vi "Update CW Indicators.vi"(8 "error  in":errorcluster, 10 "Car Wash Steps":string[][](array[string]), 11 "Position Correct?":bool) -> (0 "error out":errorcluster, 3 "Car Wash Indicators":T1)   [LabVIEW 2020]
uses:
  Controls/Car Wash Indicators.ctl
  7d301b4d-829d-4e45-9de8-334e8fe51d28.vi
  <vilib>/Comparison/Equal/Equal Functor/Equal Functor.lvclass
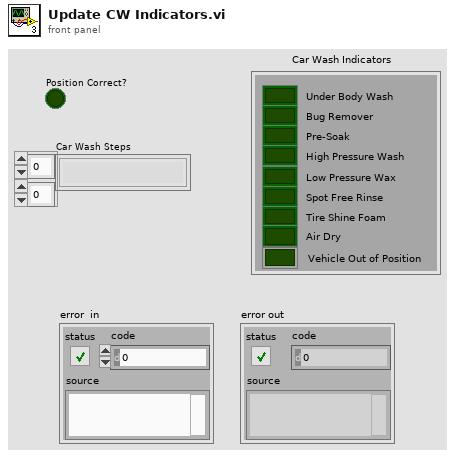
[diagram p1: front panel]
types:
  T1 = typedef "Car Wash Indicators.ctl" = cluster{"Under Body Wash":bool, "Bug Remover":bool, "Pre-Soak":bool, "High Pressure Wash":bool, "Low Pressure Wax":bool, "Spot Free Rinse":bool, "Tire Shine Foam":bool, "Air Dry":bool, "Vehicle Out of Position":bool}
  T2 = cluster{"Car Wash Indicators[0]":bool, "Car Wash Indicators[1]":bool, "Car Wash Indicators[2]":bool, "Car Wash Indicators[3]":bool, "Car Wash Indicators[4]":bool, "Car Wash Indicators[5]":bool, "Car Wash Indicators[6]":bool, "Car Wash Indicators[7]":bool, "Car Wash Indicators[8]":bool}
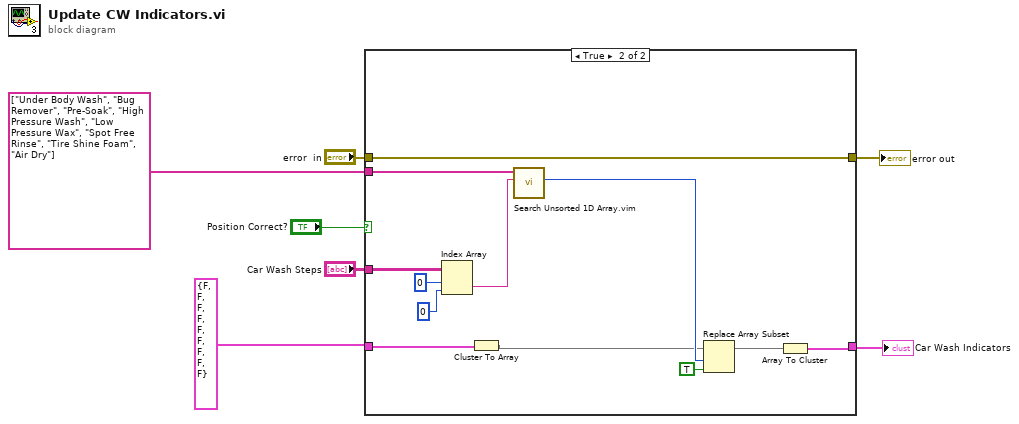
[diagram p0: block diagram]
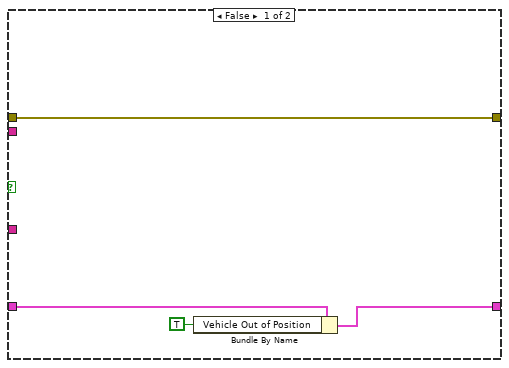
[diagram p2: hidden frame]
diagram:
  n1 = case shown="True" "Position Correct?" {
    tunnel: string[] ["Under Body Wash", "Bug Remover", "Pre-Soak", "High Pressure Wash", "Low Pressure Wax", "Spot Free Rinse", "Tire Shine Foam", "Air Dry"] ("Array") -> [_ w21]
    tunnel: T1 {"Under Body Wash"=FALSE, "Bug Remover"=FALSE, "Pre-Soak"=FALSE, "High Pressure Wash"=FALSE, "Low Pressure Wax"=FALSE, "Spot Free Rinse"=FALSE, "Tire Shine Foam"=FALSE, "Air Dry"=FALSE, "Vehicle Out of Position"=FALSE} ("Car Wash Indicators") -> [w10 w16]
    tunnel: [w8 w19] -> w7
    tunnel: "error  in" -> [w11 w14]
    tunnel: [w11 w14] -> w4
    tunnel: "Car Wash Steps" -> [_ w12]
    frame False {
      n2 = Bundle By Name(cluster=w10, "Vehicle Out of Position"=TRUE) -> (w8:T1)
    }
    frame True {
      n3 = Index Array(array=w12, index (row)=0, index (col)=0 ("disabled index (col)")) -> (element=w20:string)
      n4 = Cluster To Array(cluster=w16) -> (array=w15:bool[])
      n5 = call "Search Unsorted 1D Array.vim"("element"=w20, "unsorted 1D array"=w21) -> ("index of element"=w17:i32)  [unwired: 9 in]
      n6 = Replace Array Subset(array=w15, new element=TRUE ("new element/subarray"), index=w17) -> (w18:bool[])
      n7 = Array To Cluster(array=w18) -> (cluster=w19:T2)
    }
  }
  "Car Wash Indicators" <- w7
  "error out" <- w4
